vi "Table_FormatLimitsTemplate.vi"(8 "error in (no error)":errorcluster, 11 "Selections":string[][](array[string])) -> (0 "error out":errorcluster, 3 "Data":string[](array[string]))   [LabVIEW 2012, in "TableSupportLib.lvlib"]
uses:
  TableSupportLib.lvlib
  Table_Globals.vi
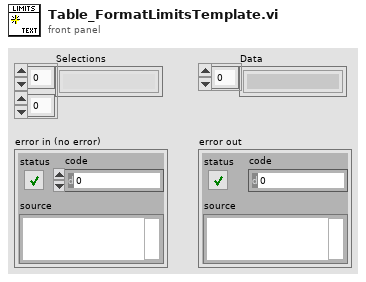
[diagram p1: front panel]
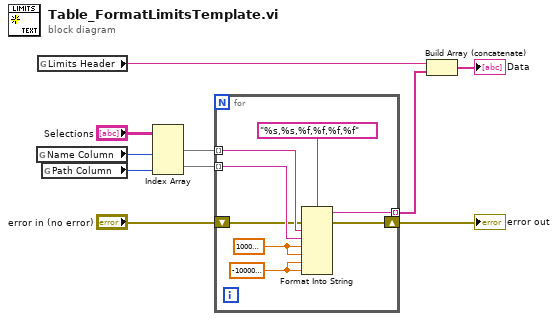
[diagram p0: block diagram]
diagram:
  n1 = global read "Table_Globals.vi" "Name Column"() -> (w5:i32)
  n2 = global read "Table_Globals.vi" "Limits Header"() -> (w9:string)
  n3 = global read "Table_Globals.vi" "Path Column"() -> (w4:i32)
  n4 = Index Array(array="Selections", index (col) #1=w5, index (col) #2=w4) -> (element #1=w3:string[], element #2=w6:string[])  [unwired: 2 in]
  n5 = for {
    shift-right: [w16] -> w7
    shift-left: "error in (no error)" -> [w13]
    tunnel: w3 -> [w18] mode=indexing
    tunnel: w6 -> [w17] mode=indexing
    tunnel: [w15] -> w8 mode=indexing
    w11 = -10000000000.0
    w12 = 10000000000.0
    n6 = Format Into String(format string="%s,%s,%f,%f,%f,%f", error in=w13, w18, w17, w12, w12, w11, w11) -> (resulting string=w15:string, error out=w16:errorcluster)  [unwired: 1 in]
  }
  "error out" <- w7
  n7 = Build Array (concatenate)(w9, w8) -> (→"Data":string[])
